vi "GUI.Comprueba limites.vi"(1 "LIMITS MEASUREMENT ADC":string[][](array[string]), 2 "LIMITS MEASUREMENT ADC 2":string[][](array[string])) -> (0 "Array":string[][](array[string]))   [LabVIEW 2019]
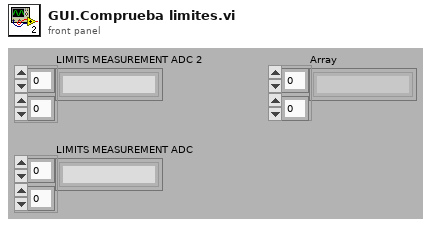
[diagram p1: front panel]
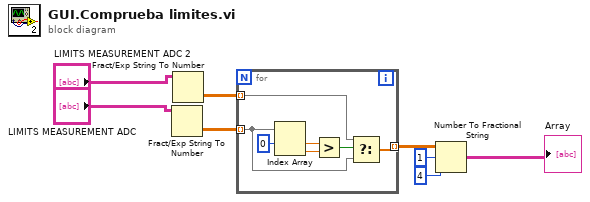
[diagram p0: block diagram]
diagram:
  n1 = Fract/Exp String To Number(string="LIMITS MEASUREMENT ADC") -> (number=w3:dbl[][])  [unwired: 3 in, 1 out]
  n2 = Fract/Exp String To Number(string="LIMITS MEASUREMENT ADC 2") -> (number=w2:dbl[][])  [unwired: 3 in, 1 out]
  n3 = for {
    tunnel: w3 -> [w9] mode=indexing
    tunnel: w2 -> [w10] mode=indexing
    tunnel: [w11] -> w1 mode=indexing
    n4 = Index Array(array=w9, index #1=0 ("index")) -> (element #1=w13:dbl, element #2=w14:dbl)  [unwired: 1 in]
    n5 = Greater?(x=w13, y=w14) -> (0:w12:bool)
    n6 = Select(t=w10, s=w12, f=w9) -> (s? t:f=w11:dbl[])
  }
  n7 = Number To Fractional String(number=w1, width (-)=i16 1, precision (6)=i16 4) -> (F-format string=→"Array":string[][])  [unwired: 1 in]
